vi "Convert File (Track) Name to File Path.vi"(11 "Track Names":T2) -> (3 "Track File Paths":T1)   [LabVIEW 2015]
doc: "Creates an appropriate File Path for given file (track) names."
uses:
  Controls/Track File Names.ctl
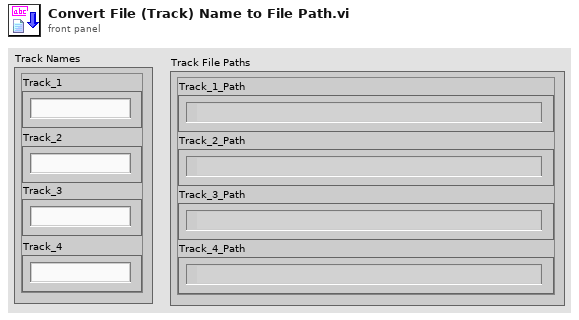
[diagram p1: front panel]
types:
  T1 = cluster{"Track_1_Path":path, "Track_2_Path":path, "Track_3_Path":path, "Track_4_Path":path}
  T2 = typedef "Track File Names.ctl" = cluster{"Track_1":string, "Track_2":string, "Track_3":string, "Track_4":string}
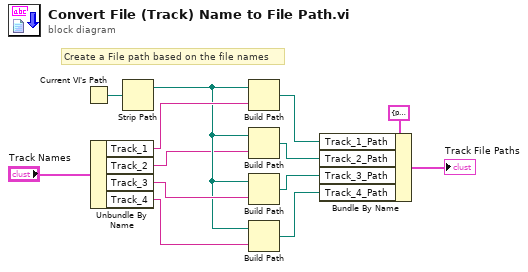
[diagram p0: block diagram]
diagram:
  # "Create a File path based on the file names"
  n1 = Current VI's Path() -> (path=w13:path)
  n2 = Unbundle By Name("Track Names") -> ("Track_1"=w11:string, "Track_2"=w7:string, "Track_3"=w10:string, "Track_4"=w9:string)
  n3 = Strip Path(path=w13) -> (stripped path=w8:path)  [unwired: 1 out]
  n4 = Build Path(base path=w8, name or relative path=w11) -> (appended path=w6:path)
  n5 = Build Path(base path=w8, name or relative path=w7) -> (appended path=w4:path)
  n6 = Build Path(base path=w8, name or relative path=w10) -> (appended path=w3:path)
  n7 = Build Path(base path=w8, name or relative path=w9) -> (appended path=w2:path)
  n8 = Bundle By Name(cluster=T1 {"Track_1_Path"=path "", "Track_2_Path"=path "", "Track_3_Path"=path "", "Track_4_Path"=path ""}, "Track_1_Path"=w6, "Track_2_Path"=w4, "Track_3_Path"=w3, "Track_4_Path"=w2) -> (→"Track File Paths":T1)
